vi "PROBE (To String).vi"(11 "Carya Config.lvclass":refnum<class "Carya Config.lvclass">) -> (2 "Value String":string, 3 "Boolean":bool)   [LabVIEW 2013, in "Carya Config.lvclass"]
doc: "Copyright 2018, Carya Automatisering, Wiebe Walstra."
uses:
  Carya Config.lvclass
panel:
  out "String":string
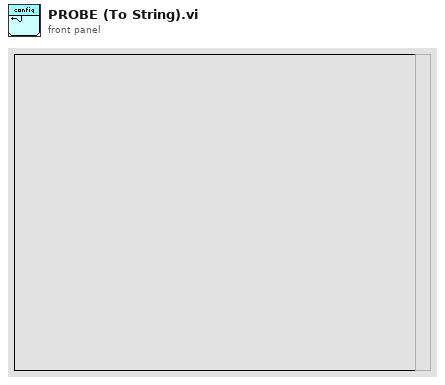
[diagram p1: front panel]
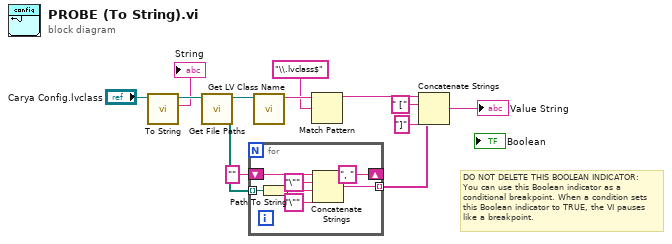
[diagram p0: block diagram]
diagram:
  # "DO NOT DELETE THIS BOOLEAN INDICATOR: \nYou can use this Boolean indicator as a conditional breakpoint. When a condition sets this Boolean indicator to TRUE, the VI pauses like a breakpoint."
  n1 = call-dynamic "To String.vi"("Carya Config in"="Carya Config.lvclass") -> ("String"=→"String":string, "Carya Config out"=w2:refnum<class "Carya Config.lvclass">)  [unwired: 8 in, 1 out]
  n2 = call-dynamic "Get File Paths.vi"("Carya Config in"=w2) -> ("Paths (all)"=w6:path[], "Carya Config out"=w13:refnum<class "Carya Config.lvclass">)  [unwired: 7 in, 2 out]
  n3 = for {
    tunnel: w6 -> [w20] mode=indexing
    shift-right: [", " ("string")] -> _
    shift-left: "" ("string") -> [w16]
    tunnel: [w15] -> w5 mode=indexing
    n4 = Path To String(path=w20) -> (string=w17:string)
    n5 = Concatenate Strings(w16, "\"" ("string"), w17, "\"" ("string")) -> (w15:string)
  }
  n6 = call <vilib>:"Get LV Class Name.vi"("object"=w13) -> ("class name"=w12:string)  [unwired: 9 in, 1 out]
  n7 = Match Pattern(string=w12, regular expression="\\.lvclass$") -> (before substring=w10:string)  [unwired: 1 in, 3 out]
  n8 = Concatenate Strings(w10, " [" ("string"), w5, "]" ("string")) -> (→"Value String":string)
